vi "Unicode Text File Example.vi"() -> ()   [LabVIEW 2020]
doc: "This example demonstrates reading and displaying unicode text from a file."
uses:
  6e33b54d-a1f2-45fa-88c6-036dd802949b.vi
  Types/UTF-8 String/UTF-8 String.lvclass
  G-Unicode.lvlib
  Unicode/Controls/String Encoding.ctl
  Types/UTF-8 Path/UTF-8 Path.lvclass
  Dialog & User Interface/Polymorphic VIs/Write Control Text/Write String Value (UTF-8 String).vi
  45627e68-18eb-4edc-9747-f3175908f235.vi
panel:
  out "Raw File Contents":string
  out "Detected Encoding":T1
  out "Encoded File Contents":string
  out "Path":string
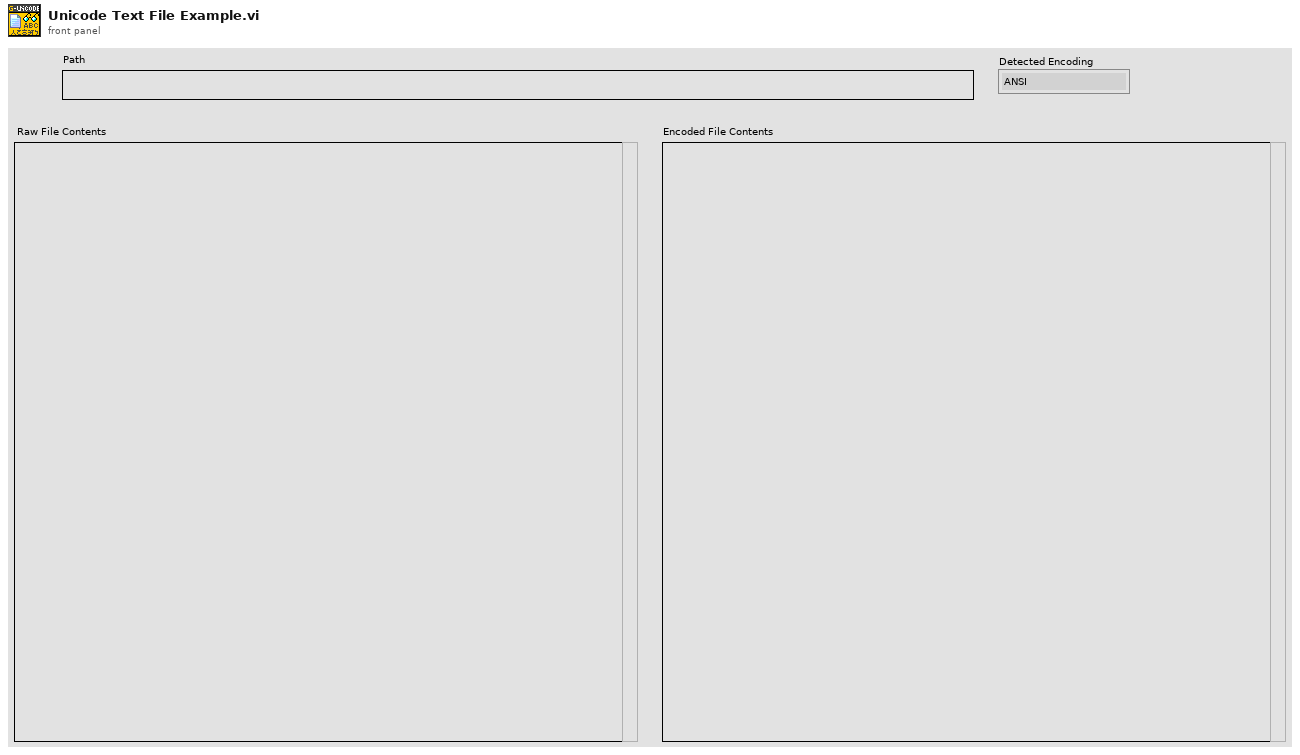
[diagram p1: front panel]
types:
  T1 = typedef "G-Unicode.lvlib/String Encoding.ctl" = enum16{"ANSI", "UTF-8", "UTF-16LE", "UTF-16BE", "Unknown"}
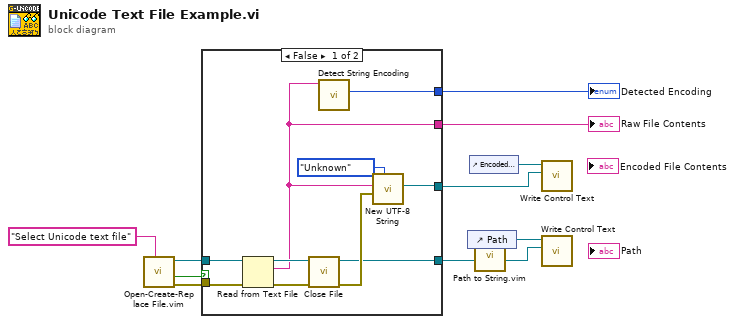
[diagram p0: block diagram]
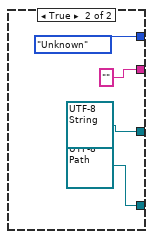
[diagram p2: hidden frame]
diagram:
  n1 = call "Open-Create-Replace File.vim"("Prompt"="Select Unicode text file") -> ("error out"=w10:errorcluster, "Cancelled"=w9:bool, "Refnum out"=w11:refnum<file>)  [unwired: 8 in]
  n2 = case shown="False" w9 {
    tunnel: w11 -> [w17 _]
    tunnel: w10 -> [w16 _]
    tunnel: [w15 String_Encoding."Unknown" ("Encoding")] -> w5
    tunnel: [w14 refnum<class "UTF-8 String.lvclass"> refnum ("UTF-8 String")] -> w4
    tunnel: [w13 refnum<class "UTF-8 Path.lvclass"> refnum ("UTF-8 Path")] -> w3
    tunnel: [w12 ""] -> w2
    frame False {
      n3 = Read from Text File(file (use dialog)=w17, error in=w16) -> (refnum out=w20:refnum<file>, text=w12:string, error out=w19:errorcluster)  [unwired: 2 in, 1 out]
      n4 = call "Close File.vi"("error in"=w19, "Refnum"=w20) -> ("error out"=w18:errorcluster, "UTF-8 Path"=w13:refnum<class "UTF-8 Path.lvclass">)  [unwired: 8 in]
      n5 = call "Detect String Encoding.vi"("String"=w12) -> ("Encoding"=w15:T1)  [unwired: 8 in, 2 out]
      n6 = call "New UTF-8 String.vi"("Input Encoding (ANSI)"=String_Encoding."Unknown", "error in"=w18, "String"=w12) -> ("UTF-8 String"=w14:refnum<class "UTF-8 String.lvclass">)  [unwired: 7 in, 1 out]
    }
    frame True {
    }
  }
  "Detected Encoding" <- w5
  "Raw File Contents" <- w2
  n7 = control-ref of="Path"() -> (w7:refnum<vi>)
  n8 = control-ref of="Encoded File Contents"() -> (w6:refnum<vi>)
  n9 = call "Path to String.vim"("Path"=w3) -> ("String"=w1:refnum<class "UTF-8 String.lvclass">)  [unwired: 9 in, 1 out]
  n10 = call-poly "Write Control Text.vi"("Value"=w4, "Control Ref"=w6) -> ()  [unwired: 9 in, 1 out]
  n11 = call-poly "Write Control Text.vi"("Value"=w1, "Control Ref"=w7) -> ()  [unwired: 9 in, 1 out]
